vi "hold_status.vi"(8 "Persistence (sec)":dbl=0.5, 10 "Update":bool, 11 "New event":T1 {"Timestamp" format="%<%.3X>T"}) -> (0 "Error":bool, 1 "Warning":bool, 3 "Hold status":T1[](array[typedef]) {"Timestamp" format="%<%.3X>T"})   [LabVIEW 2012]
uses:
  log_event.ctl
  initialization/micron_globals.vi
panel:
  # "This works in conjunction with the status aggregator loop to maintain a copy of the status where non-OK events are \"sticky\" so that transient events can be noticed."
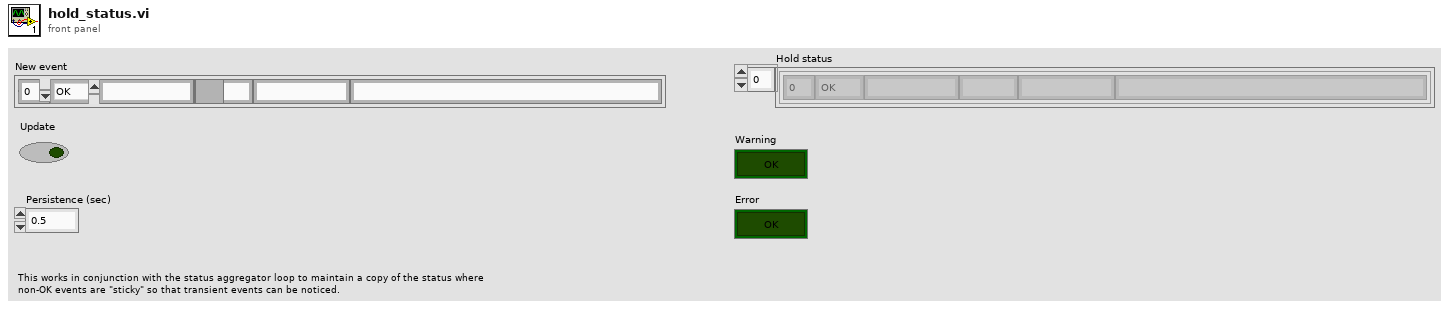
[diagram p1: front panel]
types:
  T1 = typedef "log_event.ctl" = cluster{"Facility ID":i32, "Severity":enum16{"OK", "Debug", "Warn", "Error"}, "Timestamp":timestamp, "Facility":string, "State":string, "Message":string}
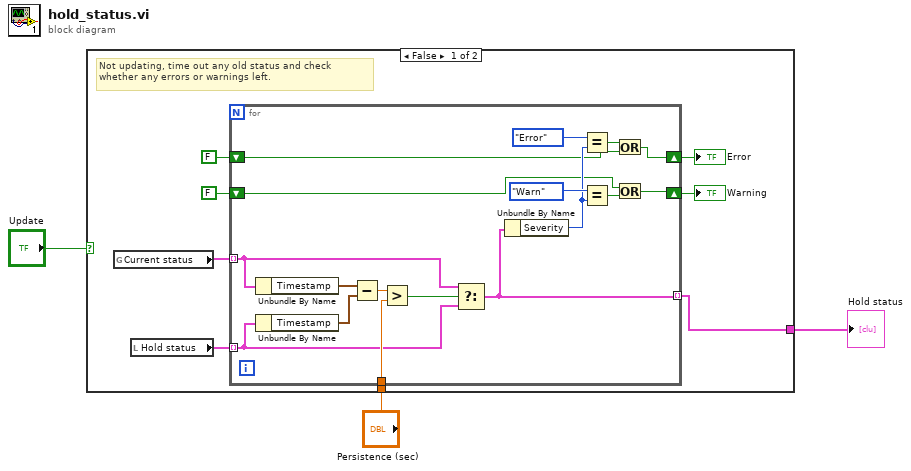
[diagram p0: block diagram]
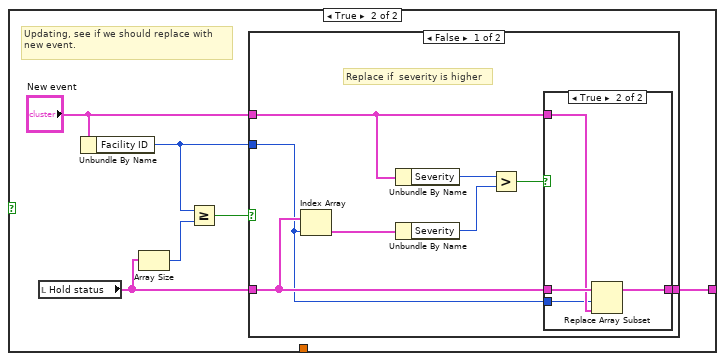
[diagram p2: hidden frame]
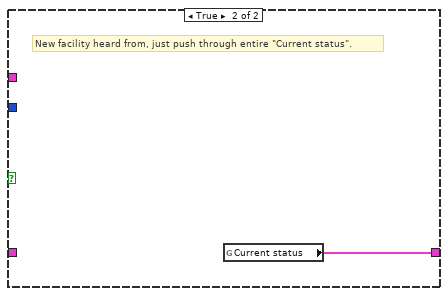
[diagram p4: hidden frame]
diagram:
  n1 = case shown="False" "Update" {
    tunnel: [w4 w29] -> w2
    tunnel: "Persistence (sec)" -> [w5 _]
    frame False {
      # "Not updating, time out any old status and check whether any errors or warnings left."
      n2 = global read "micron_globals.vi" "Current status"() -> (w6:T1[])
      n3 = local read "Hold status"() -> (w7:T1[])
      n4 = for {
        shift-right: [w20] -> w10
        shift-left: FALSE -> [w21]
        shift-right: [w24] -> w11
        shift-left: FALSE -> [w23]
        tunnel: w7 -> [w13] mode=indexing
        tunnel: w6 -> [w14] mode=indexing
        tunnel: w5 -> [w16]
        tunnel: [w12] -> w4 mode=indexing
        n5 = Unbundle By Name(w14) -> ("Timestamp"=w17:timestamp)
        n6 = Unbundle By Name(w13) -> ("Timestamp"=w18:timestamp)
        n7 = Subtract(x=w17, y=w18) -> (x-y=w19:dbl)
        n8 = Greater?(x=w19, y=w16) -> (0:w15:bool)
        n9 = Select(t=w14, s=w15, f=w13) -> (s? t:f=w12:T1)
        n10 = Unbundle By Name(w12) -> ("Severity"=w26:enum16{"OK", "Debug", "Warn", "Error"})
        n11 = Equal?(x=enum16{"OK", "Debug", "Warn", "Error"}."Error" ("Severity"), y=w26) -> (x = y?=w22:bool)
        n12 = Equal?(x=enum16{"OK", "Debug", "Warn", "Error"}."Warn" ("Severity"), y=w26) -> (x = y?=w25:bool)
        n13 = Or(x=w22, y=w21) -> (x .or. y?=w20:bool)
        n14 = Or(x=w23, y=w25) -> (x .or. y?=w24:bool)
      }
      "Error" <- w10
      "Warning" <- w11
    }
    frame True {
      # "Updating, see if we should replace with new event."
      n15 = local read "Hold status"() -> (w30:T1[])
      n16 = Unbundle By Name("New event") -> ("Facility ID"=w32:i32)
      n17 = Array Size(array=w30) -> (size(s)=w34:i32)
      n18 = Greater Or Equal?(x=w32, y=w34) -> (x >= y?=w31:bool)
      n19 = case shown="False" w31 {
        tunnel: "New event" -> [w39 _]
        tunnel: w30 -> [w38 _]
        tunnel: w32 -> [w37 _]
        tunnel: [w36 w48] -> w29
        frame False {
          # "Replace if  severity is higher"
          n20 = Index Array(array=w38, index=w37) -> (element=w40:T1)
          n21 = Unbundle By Name(w39) -> ("Severity"=w41:enum16{"OK", "Debug", "Warn", "Error"})
          n22 = Unbundle By Name(w40) -> ("Severity"=w42:enum16{"OK", "Debug", "Warn", "Error"})
          n23 = Greater?(x=w41, y=w42) -> (0:w35:bool)
          n24 = case shown="True" w35 {
            tunnel: w39 -> [_ w46]
            tunnel: w38 -> [w43 w47]
            tunnel: w37 -> [_ w45]
            tunnel: [w43 w44] -> w36
            frame False {
            }
            frame True {
              n25 = Replace Array Subset(array=w47, new element=w46, index=w45) -> (w44:T1[])
            }
          }
        }
        frame True {
          # "New facility heard from, just push through entire \"Current status\"."
          n26 = global read "micron_globals.vi" "Current status"() -> (w48:T1[])
        }
      }
    }
  }
  "Hold status" <- w2
